vi "SavedSettingsRestoreVIPosition.vi"(7 "VI ref":refnum<vi>, 8 "error in (no error)":errorcluster, 9 "Value for VI":string, 10 "VI Name":string, 11 "Application in":refnum<vi>) -> (0 "error out":errorcluster)   [LabVIEW 2019]
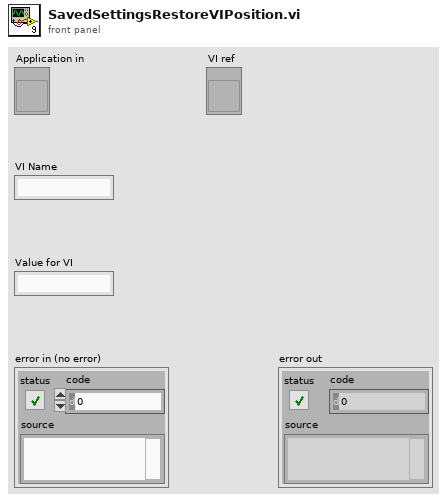
[diagram p1: front panel]
types:
  T1 = enum32{"Invalid", "Standard", "Closed", "Hidden", "Minimized", "Maximized"}
  T2 = cluster{"[0]":i32, "[1]":i32, "[2]":i32, "[3]":i32}
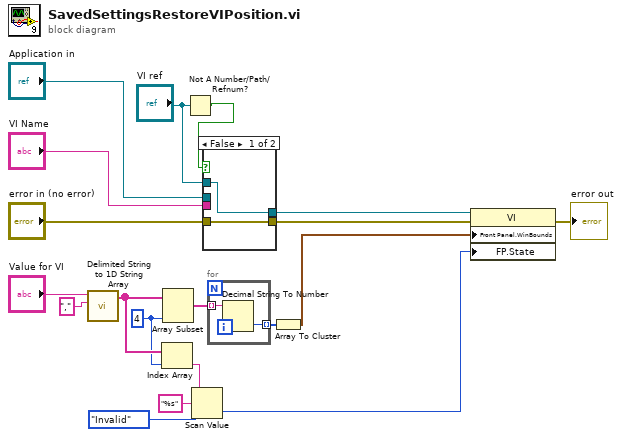
[diagram p0: block diagram]
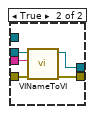
[diagram p2: hidden frame]
diagram:
  w10 = 4 ("length")
  n1 = call <vilib>:"Delimited String to 1D String Array.vi"("delimiter"=",", "delimited string"="Value for VI") -> ("string array"=w11:string[])  [unwired: 9 in]
  n2 = Index Array(array=w11, index=w10) -> (element=w6:string)
  n3 = Array Subset(array=w11, length=w10) -> (w9:string[])  [unwired: 1 in]
  n4 = Not A Number/Path/Refnum?(number/path/refnum="VI ref") -> (NaN/Path/Refnum?=w2:bool)
  n5 = Scan Value(string=w6, format string="%s", default (0 dbl)=T1."Invalid" ("Front Panel Window:State")) -> (value=w3:T1)  [unwired: 1 out]
  n6 = case shown="False" w2 {
    tunnel: [w20 w26] -> w18
    tunnel: [w21 w25] -> w17
    tunnel: "error in (no error)" -> [w20 w24]
    tunnel: "VI Name" -> [_ w23]
    tunnel: "Application in" -> [_ w22]
    tunnel: "VI ref" -> [w21 _]
    frame False {
    }
    frame True {
      n7 = call "VINameToVI.vi"("error in (no error)"=w24, "vi"=w23, "Application in"=w22) -> ("error out"=w26:errorcluster, "VI out"=w25:refnum<vi>)  [unwired: 7 in]
    }
  }
  n8 = for {
    tunnel: w9 -> [w28] mode=indexing
    tunnel: [w27] -> w8 mode=indexing
    n9 = Decimal String To Number(string=w28) -> (number=w27:i32)  [unwired: 2 in, 1 out]
  }
  n10 = Array To Cluster(array=w8) -> (cluster=w7:T2)
  n11 = property class="VI"(reference=w17, error in=w18, "Front Panel.WinBounds"=w7, "FP.State"=w3) -> (error out=→"error out":errorcluster)  [unwired: 1 out]
